vi "rszvl_core_global.vi"() -> ()   [LabVIEW 2014] (continued)
"*WAI"=FALSE}, "Check Status Callback"=""}, {"Level"=2, "Descriptive Name"="Display Window Size", "Class Only"=FALSE, "Data Type"=0, "Access"=2, "Identifier"="RSZVL_ATTR_DISP_WINDOW_SIZE", "Range Table"="rszvl_rngDISPSizeWindow", "Command"="DISP:SIZE", "Read Callback"="", "Write Callback"="", "Range Callback"="", "Check Callback"="", "Rngtable Callback"="", "Coerce Callback"="", "User Callback"="", "Supported Models"="", "Instrument Options"="", "Repeated Capabilities"="", "Restricted Repeated Capabilities"="", "Help"="This attribute switches the measurement window for channel and adjacent-channel power measurements to full screen or half screen.\n\nAvailable Repeated Capabilities:\nNone\n\nRemote-control command(s):\nDISPlay[:WINDow<1|2>]:SIZE LARGe | SMALl", "Flags"={"OPC Wait"=FALSE, "Dont check status"=FALSE, "*WAI"=FALSE}, "Check Status Callback"=""}, {"Level"=2, "Descriptive Name"="Display Color Preset", "Class Only"=FALSE, "Data Type"=4, "Access"=1, "Identifier"="RSZVL_ATTR_DISP_COL_PRESET", "Range Table"="", "Command"="DISP:CMAP:DEF{Default}", "Read Callback"="", "Write Callback"="", "Range Callback"="", "Check Callback"="", "Rngtable Callback"="", "Coerce Callback"="", "User Callback"="", "Supported Models"="", "Instrument Options"="", "Repeated Capabilities"="", "Restricted Repeated Capabilities"="", "Help"="This attribute resets the screen colors of all display items to their default settings. Two default settings DEFault1 and DEFault2 are available. The numeric suffix of CMAP is irrelevant.\n\nAvailable Repeated Capabilities:\nDefault: DEF1,DEF2,DEF3\r\n\nRemote-control command(s):\nDISPlay:CMAP<1 to 27>:DEFault<1|2|3>", "Flags"={"OPC Wait"=FALSE, "Dont check status"=FALSE, "*WAI"=FALSE}, "Check Status Callback"=""}, {"Level"=2, "Descriptive Name"="Display Color Predefined", "Class Only"=FALSE, "Data Type"=0, "Access"=1, "Identifier"="RSZVL_ATTR_DISP_COL_PREDEFINED", "Range Table"="rszvl_rngDISPConfPreDefColour", "Command"="DISP:CMAP{CMAP}:PDEF", "Read Callback"="", "Write Callback"="", "Range Callback"="", "Check Callback"="", "Rngtable Callback"="", "Coerce Callback"="", "User Callback"="", "Supported Models"="", "Instrument Options"="", "Repeated Capabilities"="", "Restricted Repeated Capabilities"="", "Help"="This attribute defines the color table of the instrument using predefined color values. Each numeric suffix of CMAP is assigned one or several graphical elements which can be modified by varying the corresponding color setting.\nThe same assignment as for DISPlay:CMAP<1 to 26>:HSL applies.\n\nAvailable Repeated Capabilities:\nCMAP: CM1,CM2,CM3,CM4,CM5,CM6,CM7,CM8,CM9,CM10,CM11,CM12,CM13,CM14,CM15,CM16,CM17,CM18,CM19,CM20,CM21,CM22,CM23,CM24,CM25,CM26,CM27\r\n\nRemote-control command(s):\nDISPlay:CMAP<1 to 27>:PDEFined BLACk| BLUE| BROWn| GREen|MAGenta| YELLow| WHITe| DGRAy| LGRAy|LBLUe| LGREen| LCYan| LRED| MAGenta", "Flags"={"OPC Wait"=FALSE, "Dont check status"=FALSE, "*WAI"=FALSE}, "Check Status Callback"=""}, {"Level"=2, "Descriptive Name"="Display Log Range", "Class Only"=FALSE, "Data Type"=1, "Access"=2, "Identifier"="RSZVL_ATTR_DISP_LOG_RANGE", "Range Table"="rszvl_rngDISPAmplitudeRang", "Command"="DISP:WIND:TRAC:Y", "Read Callback"="", "Write Callback"="", "Range Callback"="", "Check Callback"="", "Rngtable Callback"="", "Coerce Callback"="", "User Callback"="", "Supported Models"="", "Instrument Options"="", "Repeated Capabilities"="", "Restricted Repeated Capabilities"="", "Help"="This attribute defines the display range of the Y axis (level axis) with logarithmic scaling (DISP:TRAC:Y:SPAC LOG).\nFor linear scaling, (DISP:TRAC:Y:SPAC LIN | PERC) the display range is fixed and cannot be modified.\n\nAvailable Repeated Capabilities:\nNone\n\nRemote-control command(s):\nDISPlay[:WINDow<1|2>]:TRACe<1 to 6>:Y[:SCALe]", "Flags"={"OPC Wait"=FALSE, "Dont check status"=FALSE, "*WAI"=FALSE}, "Check Status Callback"=""}, {"Level"=2, "Descriptive Name"="Display Amplitude Grid Mode", "Class Only"=FALSE, "Data Type"=0, "Access"=2, "Identifier"="RSZVL_ATTR_DISP_AMPLITUDE_GRID_MODE", "Range Table"="rszvl_rngAbsRel", "Command"="DISP:WIND:TRAC:Y:MODE", "Read Callback"="", "Write Callback"="", "Range Callback"="", "Check Callback"="", "Rngtable Callback"="", "Coerce Callback"="", "User Callback"="", "Supported Models"="", "Instrument Options"="", "Repeated Capabilities"="", "Restricted Repeated Capabilities"="", "Help"="This attribute defines the scale type of the Y axis (absolute or relative).\nWhen SYSTem:DISPlay is set to OFF, this command has no immediate effect on the screen. The numeric suffix is irrelevant.\n\nAvailable Repeated Capabilities:\nNone\n\nRemote-control command(s):\nDISPlay[:WINDow<1|2>]:TRACe<1 to 6>:Y[:SCALe]:MODE ABSolute | RELative", "Flags"={"OPC Wait"=FALSE, "Dont check status"=FALSE, "*WAI"=FALSE}, "Check Status Callback"=""}, {"Level"=2, "Descriptive Name"="Display During Single Sweep", "Class Only"=FALSE, "Data Type"=3, "Access"=2, "Identifier"="RSZVL_ATTR_DISP_SINGLE_SWEEP", "Range Table"="", "Command"="INIT:DISP", "Read Callback"="", "Write Callback"="", "Range Callback"="", "Check Callback"="", "Rngtable Callback"="", "Coerce Callback"="", "User Callback"="", "Supported Models"="", "Instrument Options"="", "Repeated Capabilities"="", "Restricted Repeated Capabilities"="", "Help"="This attribute configures the behaviour of the display during a single sweep.\nINITiate:DISPlay OFF means that the display is switched off during the measurement, INITiate:DISPlay ON means that the display is switched on during the measurement.\n\nAvailable Repeated Capabilities:\nNone\n\nRemote-control command(s):\nINITiate:DISPlay ON | OFF", "Flags"={"OPC Wait"=FALSE, "Dont check status"=FALSE, "*WAI"=FALSE}, "Check Status Callback"=""}, {"Level"=2, "Descriptive Name"="Display Update", "Class Only"=FALSE, "Data Type"=3, "Access"=2, "Identifier"="RSZVL_ATTR_DISP_UPDATE", "Range Table"="", "Command"="SYST:DISP:UPD", "Read Callback"="", "Write Callback"="", "Range Callback"="", "Check Callback"="", "Rngtable Callback"="", "Coerce Callback"="", "User Callback"="", "Supported Models"="", "Instrument Options"="", "Repeated Capabilities"="", "Restricted Repeated Capabilities"="", "Help"="This attribute switches on or off the update of all display elements during remote control.\n\nNote: \n(1) The best performance is obtained when the display output is switched off during remote control.\n\nAvailable Repeated Capabilities:\nNone\n\nRemote-control command(s):\nSYSTem:DISPlay:UPDate ON | OFF", "Flags"={"OPC Wait"=FALSE, "Dont check status"=FALSE, "*WAI"=FALSE}, "Check Status Callback"=""}, {"Level"=2, "Descriptive Name"="Configure Display Unit Power", "Class Only"=FALSE, "Data Type"=0, "Access"=2, "Identifier"="RSZVL_ATTR_UNIT_POWER", "Range Table"="rszvl_rngAmplitudeUnitsRangeTable", "Command"="CALC:UNIT:POW", "Read Callback"="", "Write Callback"="", "Range Callback"="", "Check Callback"="", "Rngtable Callback"="", "Coerce Callback"="", "User Callback"="", "Supported Models"="", "Instrument Options"="", "Repeated Capabilities"="", "Restricted Repeated Capabilities"="", "Help"="This attribute selects the unit for power.\n\nAvailable Repeated Capabilities:\nNone\n\nRemote-control command(s):\nCALCulate<1|2>:UNIT:POWer DBM | V | A | W | DBPW | WATT | DBUV | DBMV | VOLT | DBUA | AMPere |DBUV_M | DBUA_M", "Flags"={"OPC Wait"=FALSE, "Dont check status"=FALSE, "*WAI"=FALSE}, "Check Status Callback"=""}, {"Level"=1, "Descriptive Name"="Markers", "Class Only"=TRUE, "Data Type"=0, "Access"=0, "Identifier"="", "Range Table"="", "Command"="", "Read Callback"="", "Write Callback"="", "Range Callback"="", "Check Callback"="", "Rngtable Callback"="", "Coerce Callback"="", "User Callback"="", "Supported Models"="", "Instrument Options"="", "Repeated Capabilities"="", "Restricted Repeated Capabilities"="", "Help"="(1) Marker Amplitude:\nThis attribute queries the measured value of the selected marker. The corresponding marker is activated before or switched to marker mode, if necessary.\nTo obtain a valid query result, a complete sweep with synchronization to the sweep end must be performed between the activation of the marker and the query of the y value. This is only possible in single sweep mode.\nThe query result is output in the unit determined with CALCulate:UNIT.\n\n(2) Marker State:\nThis attribute switches on or off the currently selected marker. If no indication is made, marker 1 is selected automatically. If marker 2, 3 or 4 is selected and used as a delta marker, it is switched to marker mode.\n\n(3) Marker Position:\nThis attribute positions the selected marker to the indicated frequency (span > 0), time (span = 0) or level (APD measurement or CCDF measurement ON). If marker 2, 3 or 4 is selected and used as delta marker, it is switched to marker mode.\n\n(4) Assign Marker to Trace:\nThis attribute assigns the selected marker to the indicated measurement curve. The corresponding trace must be active, i.e. its status must be different from BLANK.\n\n(5) All Markers Off:\nThis attribute switches off all active markers.\n\n(6) Marker Local Oscillator Suppression:\nThis attribute switches the local oscillator suppression for peak search on or off. This setting is valid for all markers and delta markers.\n\n(7) Signal Track State:\nThis attribute switches the signal-track function on or off. The function is independent of the selected marker.\nWith signal track activated, the maximum signal is determined after each frequency sweep and the center frequency is set to the frequency of this signal. Thus with drifting signals the center frequency follows the signal.\n\n(8) Signal Track Bandwidth:\nThis attribute defines the bandwidth around the center frequency within which the largest signal is searched. It is only available in the frequency domain (span > 0).\n\nNote(s):\n(1) The entry of the search bandwidth is only possible if the Signal Track function is switched on (RSZVL_ATTR_SIGNAL_TRACK_STATE).\n\n(9) Signal Track Threshold:\nThis attribute defines the threshold above which the largest signal is searched for. The function is independent of the selected marker. It is only available in the frequency domain (span > 0).\nThe response unit depends on the settings defined with CALC:UNIT.\n\nNote(s):\n(1) The entry of the search threshold is only possible if the Signal Track function is switched on (RSZVL_ATTR_SIGNAL_TRACK_STATE).\n\n(10) Signal Track Trace:\nThis attribute defines the trace on which the largest signal is searched for. The function is independent of the selected marker. It is only available in the frequency domain (span > 0).\n\n(11) Marker Step Size:\nThis command defines the step size of the rotary knob for marker or delta marker value changes. It takes only effect in manual operation. It is available for all base unit measurements with the exception of statistics.\n\n(12) Marker Probability:\nThis command positions the selected marker to the given probability.\n\nNote(s): \n(1) The command is only available with the CCDF measurement switched on. The associated level value can be determined with the CALCulate<1|2>:MARKer<1...4>:X command.\n\n\n(13) Marker Search (Class):\nMarker Search.\n\n(1) Marker Search Right Minimum:\nThis attribute positions the marker to the next higher minimum value to the right of the current value (i.e. in ascending X direction) on the corresponding trace.\n\n(2) Marker Search Left Minimum:\nThis attribute positions the marker to the next higher minimum value to the left of the current value (i.e. in descending X direction) on the corresponding trace.\n\n(3) Marker Search Peak Maximum:\nThis attribute positions the marker to the current maximum value of the corresponding trace. The corresponding marker is activated first or switched to the marker mode.\nNote: If no maximum value is found on the trace (level spacing to adjacent values < peak excursion), an execution error (error eode: -200) is produced.\n\n(4) Marker Search Peak Next Maximum:\nThis attribute positions the marker to the next smaller maximum value of the corresponding trace.\n\n(5) Marker Search Peak Right Maximum:\nThis attribute positions the marker to the next smaller maximum value to the right of the current value (i.e. in ascending X values) on the corresponding trace.\n\n(6) Marker Search Peak Left Maximum:\nThis attribute positions the marker to the next smaller maximum value to the left of the current value (i.e. in descending X values) on the trace.\n\n(7) Marker Search Peak Minimum:\nThis attribute positions the marker to the current minimum value of the corresponding trace. The corresponding marker is activated first or switched to marker mode, if necessary.\n\n(8) Marker Search Next Minimum:\nThis attribute positions the marker to the next higher minimum value of the corresponding trace.\n\n(9) Marker Search Peak Maximum Auto:\nThis attribute switches an automatic maximum peak search for marker 1 at the end of each particular sweep on and off. The actual marker search limit settings (LEFT LIMIT, RIGHT LIMIT, THRESHOLD, EXCLUDE LO) are taken into account.\n\n(10) Marker Search Minimum Auto:\nThis attribute switches an automatic minimum peak search for marker 1 at the end of each particular sweep on and off. The actual marker search limit settings (LEFT LIMIT, RIGHT LIMIT, THRESHOLD, EXCLUDE LO) are taken into account.\n\n(14) Marker Search Configuration (Class):\nConfigures marker search parameters.\n\n(1) Marker Threshold State:\nThis attribute switches on or off the threshold line. The unit depends on the setting performed with CALC:UNIT.\n\n(2) Marker Threshold:\nThis attribute defines the threshold value for the maximum/minimum search of markers with marker search functions MAX PEAK, NEXT PEAK, etc. The associated display line is automatically switched on.\n\n(3) Marker Peak Excursion:\nThis attribute defines the peak excursion., i.e. the spacing below a trace maximum which must be attained before a new maximum is recognized, or the spacing above a trace minimum which must be attained before a new minimum is recognized. The set value is valid for all markers and delta markers. The unit depends on the selected operating mode.\n\n(4) Marker Search Limits State:\nThis attribute switches between a limited (ON) and unlimited (OFF) search range. The function is independent of the selection of a marker.\n\n(5) Marker Search Limits Left:\nThis attribute sets the left limit of the search range for markers and delta markers. Depending on the x axis domain the indicated value defines a frequency (span > 0) or time (span = 0). The function is independent of the selection of a marker.\n\n(6) Marker Search Limits Right:\nThis attribute sets the right limit of the search range for markers and delta markers. Depending on the x axis domain the indicated value defines a frequency (span > 0) or time (span = 0). The function is independent of the selection of a marker.\n\n\n\n(15) Marker Functions (Class):\nMarker Functions.\n\n(1) Marker Peak List Count:\nThis attribute searches the selected trace for the indicated number of maxima. The number of maxima found depends on the waveform and value set for the Peak Excursion parameter, however, a maximum number of 50 maxima are determined. Only the signals which exceed their surrounding values at least by the value indicated by the peak excursion parameter will be recognized as maxima. Therefore, the number of maxima found is not automatically the same as the number of maxima desired.\n\n(2) Marker Peak List Found:\nThis attribute reads out the number of maxima found during the search. If no search for maxima has been performed, 0 is returned.\n\n(3) Marker Peak List Sort:\nThis attribute sets the sort mode for the search for maxima.\n\n(4) Marker Zoom:\nThis attribute defines the range to be zoomed around marker 1. Marker 1 is activated first, if necessary.\nThe subsequent frequency sweep is stopped at the marker position and the frequency of the signal is counted. This frequency becomes the new center frequency, and the zoomed span is set. In order to recognize the end of the operation the synchronization to the sweep end should be activated. This is only possible in single sweep mode.\n\n(5) Marker Demodulation State:\nThis attribute switches on or off the audio demodulator when the indicated marker is reached. In the frequency domain (span > 0) the hold time can be defined at the corresponding marker position with RSZVL_ATTR_MARKER_DEMOD_HOLDOFF.\nIn the time domain (span = 0) the demodulation is permanently active.\n\n(6) Marker Demodulation Type:\nThis attribute selects the demodulation type for the audio demodulator.\n\n(7) Marker Demodulation Holdoff:\nThis attribute defines the hold time at the marker position for the demodulation in the frequency domain (span > 0).\n\n(8) Marker Demodulation Continuous:\nThis attribute switches on or off the continuous demodulation in the frequency domain (span >0). Thus acoustic monitoring of the signals can be performed in the frequency domain. The function does not depend on the selected marker.\n\n(9) Marker To Center:\nThis attribute sets the center frequency equal to the frequency of the indicated marker.\nIf marker 2, 3 or 4 is selected and used as delta marker, it is switched to the marker mode.\n\n(10) Marker To Step Width:\nThis attribute sets the step width of the center frequency to the X value of the current marker. If marker 2, 3 or 4 is selected and used as delta marker, it is switched to the marker mode.\n\n(11) Marker To Reference:\nThis attribute sets the reference level to the power measured by the indicated marker. If marker 2, 3 or 4 is selected and used as delta marker, it is switched to marker mode.\n\n(12) Marker Fixed Reference State:\nThis attribute switches the relative measurement to a fixed reference value on or off. Marker 1 will be activated previously and a peak search will be performed, if necessary. If marker 1 is activated, its position becomes the reference point for the measurement. The reference point can then be modified with commands CALCulate:DELTamarker:FUNCtion:FIXed:RPOint:X and to :RPOint:Y independently of the position of marker 1 and of a trace. It is valid for all delta markers as long as the function is active.\n\n(13) Marker Fixed Ref Point Level:\nThis attribute defines a new reference point level for all delta markers for a measurement with fixed reference point.\n(CALCulate:DELTamarker:FUNCtion:FIXed:STATe ON).\nFor phase-noise measurements (CALCulate:DELTamarker:FUNCtion:PNOise:STATe ON), the command defines a new reference point level for delta marker 2.\n\n(14) Marker Fixed Ref Point Level Offset:\nThis attribute defines an additional level offset for the measurement with fixed reference value (CALCulate:DELTamarker:FUNCtion:FIXed:STATe ON). For this measurement, the offset is included in the display of all delta markers.\nFor phase-noise measurements (CALCulate:DELTamarker:FUNCtion:PNOise:STATe ON), the command defines an additional level offset which is included in the display of delta marker 2.\n\n(15) Marker Fixed Ref Point Frequency:\nThis attribute defines a new reference frequency (span > 0) or time (span = 0) for all delta markers for a measurement with fixed reference value (CALCulate:DELTamarker:FUNCtion:FIXed:STATe ON).\nFor phase-noise measurements (CALCulate:DELTamarker:FUNCtion:PNOise:STATe ON), the command defines a new reference frequency or time for delta marker 2.\n\n(16) Marker Fixed Ref Point Peak Search:\nThis attribute sets the reference point level for all delta markers for a measurement with fixed reference point (CALC:DELT:FUNC:FIX:STAT ON) to the peak of the selected trace.\n\n\n\n(16) Delta Marker (Class):\nDelta Marker attributes configuration.\n\n(1) Delta Marker State:\nThis attribute switches on and off the delta marker when delta marker 1 is selected. The corresponding marker becomes the delta marker when delta marker 2 to 4 is selected. If the corresponding marker is not activated, it will be activated and positioned on  the maximum of the measurement curve.\n\n(2) Delta Marker Mode:\nThis attribute switches between relative and absolute frequency input of the delta marker (or time with span = 0). It affects all delta markers.\nRepeated capabilitiy Delta Marker are used to prevent switching On Delta Marker 1, if the user uses Delta Marker 2.\n\n(3) Delta Marker Position:\nThis attribute positions the selected delta marker to the indicated frequency (span > 0), time (span = 0) or level (APD measurement = ON or CCDFmeasurement = ON). The input is in absolute values or relative to marker 1 depending on the attribute RSZVL_ATTR_REFERENCE_MARKER_MODE. If Reference Fixed measurement (CALCulate:DELTamarker:FUNCtion:FIXed:STATe ON) is active, relative values refer to the reference position are entered. The query always returns absolute values.\n\n(4) Delta Marker Relative Position:\nThis attribute queries the frequency (span > 0) or time (span = 0) of the selected delta marker relative to marker 1 or to the reference position ( for CALCulate:DELTamarker:FUNCtion:FIXed:STATe ON). The attribute activates the corresponding delta marker, if necessary.\n\n(5) Delta Marker Amplitude:\nThis attribute queries the measured value of the selected delta marker. The corresponding delta marker will be activated, if necessary. The output is always a relative value referred to marker 1 or to the reference position (reference fixed active).\n\n(6) Delta Marker Assign Trace:\nThis attribute assigns the selected delta marker to the indicated measurement curve. The selected measurement curve must be active, i.e. its state must be different from BLANK.\n\n(7) Delta Marker All Off:\nThis attribute switches off all active delta markers (screen A or screen B).\n\n(17) Delta Marker Search (Class):\nDelta marker search.\n\n(1) Delta Marker Peak:\nThis attribute positions the delta marker to the current maximum value on the measured curve. If necessary, the corresponding delta marker will be activated first.\n\n(2) Delta Marker Peak Next:\nThis attribute positions the delta marker to the next smaller maximum value on the measured curve. The corresponding delta marker will be activated first, if necessary.\n\n(3) Delta Marker Peak Next Right:\nThis attribute positions the delta marker to the next smaller maximum value to the right of the current value (i.e. ascending X values). The corresponding delta marker is activated first, if necessary.\n\n(4) Delta Marker Peak Next Left:\nThis attribute positions the delta marker to the next smaller maximum value to the left of the current value (i.e. descending X values). The corresponding delta marker will be activated first, if necessary.\n\n(5) Delta Marker Minimum:\nThis attribute positions the delta marker to the current minimum value on the measured crve. The corresponding delta marker will be activated first, if necessary.\n\n(6) Delta Marker Minimum Next:\nThis attribute positions the delta marker to the next higher minimum value of the measured curve. The corresponding delta marker will be activated first, if necessary.\n\n(7) Delta Marker Minimum Next Right:\nThis attribute positions the delta marker to the next higher minimum value to the right of the current value (i.e. ascending X values). The corresponding delta marker will be activated first, if necessary.\n\n(8) Delta Marker Minimum Next Left:\nThis attribute positions the delta marker to the next higher minimum value to the left of the current value (i.e. descending X values). The corresponding delta marker will be activated first, if necessary.", "Flags"={"OPC Wait"=FALSE, "Dont check status"=FALSE, "*WAI"=FALSE}, "Check Status Callback"=""}, {"Level"=2, "Descriptive Name"="Marker Amplitude", "Class Only"=FALSE, "Data Type"=1, "Access"=0, "Identifier"="RSZVL_ATTR_MARKER_AMPLITUDE", "Range Table"="", "Command"="CALC:MARK{Marker}:Y?", "Read Callback"="", "Write Callback"="", "Range Callback"="", "Check Callback"="", "Rngtable Callback"="", "Coerce Callback"="", "User Callback"="", "Supported Models"="", "Instrument Options"="", "Repeated Capabilities"="", "Restricted Repeated Capabilities"="", "Help"="This attribute queries the measured value of the selected marker. The corresponding marker is activated before or switched to marker mode, if necessary.\nTo obtain a valid query result, a complete sweep with synchronization to the sweep end must be performed between the activation of the marker and the query of the y value. This is only possible in single sweep mode.\nThe query result is output in the unit determined with CALCulate:UNIT.\n\nAvailable Repeated Capabilities:\nMarker: M1,M2,M3,M4\r\n\nRemote-control command(s):\nCALCulate<1|2>:MARKer<1 to 4>:Y?", "Flags"={"OPC Wait"=FALSE, "Dont check status"=FALSE, "*WAI"=FALSE}, "Check Status Callback"=""}, {"Level"=2, "Descriptive Name"="Marker State", "Class Only"=FALSE, "Data Type"=3, "Access"=2, "Identifier"="RSZVL_ATTR_MARKER_ENABLED", "Range Table"="", "Command"="CALC:MARK{Marker}", "Read Callback"="", "Write Callback"="", "Range Callback"="", "Check Callback"="", "Rngtable Callback"="", "Coerce Callback"="", "User Callback"="", "Supported Models"="", "Instrument Options"="", "Repeated Capabilities"="", "Restricted Repeated Capabilities"="", "Help"="This attribute switches on or off the currently selected marker. If no indication is made, marker 1 is selected automatically. If marker 2, 3 or 4 is selected and used as a delta marker, it is switched to marker mode.\n\nAvailable Repeated Capabilities:\nMarker: M1,M2,M3,M4\r\n\nRemote-control command(s):\nCALCulate<1|2>:MARKer<1 to 4>[:STATe]", "Flags"={"OPC Wait"=FALSE, "Dont check status"=FALSE, "*WAI"=FALSE}, "Check Status Callback"=""}, {"Level"=2, "Descriptive Name"="Marker Position", "Class Only"=FALSE, "Data Type"=1, "Access"=2, "Identifier"="RSZVL_ATTR_MARKER_POSITION", "Range Table"="", "Command"="CALC:MARK{Marker}:X", "Read Callback"="", "Write Callback"="", "Range Callback"="", "Check Callback"="", "Rngtable Callback"="", "Coerce Callback"="", "User Callback"="", "Supported Models"="", "Instrument Options"="", "Repeated Capabilities"="", "Restricted Repeated Capabilities"="", "Help"="This attribute positions the selected marker to the indicated frequency (span > 0), time (span = 0) or level (APD measurement or CCDF measurement ON). If marker 2, 3 or 4 is selected and used as delta marker, it is switched to marker mode.\n\nAvailable Repeated Capabilities:\nMarker: M1,M2,M3,M4\r\n\nRemote-control command(s):\nCALCulate<1|2>:MARKer<1 to 4>:X", "Flags"={"OPC Wait"=FALSE, "Dont check status"=FALSE, "*WAI"=FALSE}, "Check Status Callback"=""}, {"Level"=2, "Descriptive Name"="Assign Marker to Trace", "Class Only"=FALSE, "Data Type"=0, "Access"=2, "Identifier"="RSZVL_ATTR_MARKER_TRACE", "Range Table"="rszvl_rngTrace", "Command"="CALC:MARK{Marker}:TRAC", "Read Callback"="", "Write Callback"="", "Range Callback"="", "Check Callback"="", "Rngtable Callback"="", "Coerce Callback"="", "User Callback"="", "Supported Models"="", "Instrument Options"="", "Repeated Capabilities"="", "Restricted Repeated Capabilities"="", "Help"="This attribute assigns the selected marker to the indicated measurement curve. The corresponding trace must be active, i.e. its status must be different from BLANK.\n\nAvailable Repeated Capabilities:\nMarker: M1,M2,M3,M4\r\n\nRemote-control command(s):\nCALCulate<1|2>:MARKer<1 to 4>:TRACe", "Flags"={"OPC Wait"=FALSE, "Dont check status"=FALSE, "*WAI"=FALSE}, "Check Status Callback"=""}, {"Level"=2, "Descriptive Name"="All Markers Off", "Class Only"=FALSE, "Data Type"=4, "Access"=1, "Identifier"="RSZVL_ATTR_MARKER_AOFF", "Range Table"="", "Command"="CALC:MARK:AOFF", "Read Callback"="", "Write Callback"="", "Range Callback"="", "Check Callback"="", "Rngtable Callback"="", "Coerce Callback"="", "User Callback"="", "Supported Models"="", "Instrument Options"="", "Repeated Capabilities"="", "Restricted Repeated Capabilities"="", "Help"="This attribute switches off all active markers.\n\nAvailable Repeated Capabilities:\nNone\n\nRemote-control command(s):\nCALCulate<1|2>:MARKer<1 to 4>:AOFF", "Flags"={"OPC Wait"=FALSE, "Dont check status"=FALSE, "*WAI"=FALSE}, "Check Status Callback"=""}, {"Level"=2, "Descriptive Name"="Marker Local Oscillator Suppression", "Class Only"=FALSE, "Data Type"=3, "Access"=2, "Identifier"="RSZVL_ATTR_MARKER_LOEX", "Range Table"="", "Command"="CALC:MARK:LOEX", "Read Callback"="", "Write Callback"="", "Range Callback"="", "Check Callback"="", "Rngtable Callback"="", "Coerce Callback"="", "User Callback"="", "Supported Models"="", "Instrument Options"="", "Repeated Capabilities"="", "Restricted Repeated Capabilities"="", "Help"="This attribute switches the local oscillator suppression for peak search on or off. This setting is valid for all markers and delta markers.\n\nAvailable Repeated Capabilities:\nNone\n\nRemote-control command(s):\nCALCulate<1|2>:MARKer<1 to 4>:LOEXclude ON | OFF", "Flags"={"OPC Wait"=FALSE, "Dont check status"=FALSE, "*WAI"=FALSE}, "Check Status Callback"=""}, {"Level"=2, "Descriptive Name"="Signal Track State", "Class Only"=FALSE, "Data Type"=3, "Access"=2, "Identifier"="RSZVL_ATTR_SIGNAL_TRACK_ENABLED", "Range Table"="", "Command"="CALC:MARK:FUNC:STR", "Read Callback"="", "Write Callback"="", "Range Callback"="", "Check Callback"="", "Rngtable Callback"="", "Coerce Callback"="", "User Callback"="", "Supported Models"="", "Instrument Options"="", "Repeated Capabilities"="", "Restricted Repeated Capabilities"="", "Help"="This attribute switches the signal-track function on or off. The function is independent of the selected marker.\nWith signal track activated, the maximum signal is determined after each frequency sweep and the center frequency is set to the frequency of this signal. Thus with drifting signals the center frequency follows the signal.\n\nAvailable Repeated Capabilities:\nNone\n\nRemote-control command(s):\nCALCulate<1|2>:MARKer<1 to 4>:FUNCtion:STRack[:STATe] ON | OFF", "Flags"={"OPC Wait"=FALSE, "Dont check status"=FALSE, "*WAI"=FALSE}, "Check Status Callback"=""}, {"Level"=2, "Descriptive Name"="Signal Track Bandwidth", "Class Only"=FALSE, "Data Type"=1, "Access"=2, "Identifier"="RSZVL_ATTR_SIGNAL_TRACK_BWID", "Range Table"="", "Command"="CALC:MARK:FUNC:STR:BWID", "Read Callback"="", "Write Callback"="", "Range Callback"="", "Check Callback"="", "Rngtable Callback"="", "Coerce Callback"="", "User Callback"="", "Supported Models"="", "Instrument Options"="", "Repeated Capabilities"="", "Restricted Repeated Capabilities"="", "Help"="This attribute defines the bandwidth around the center frequency within which the largest signal is searched. It is only available in the frequency domain (span > 0).\n\nNote(s):\n(1) The entry of the search bandwidth is only possible if the Signal Track function is switched on (RSZVL_ATTR_SIGNAL_TRACK_STATE).\n\nAvailable Repeated Capabilities:\nNone\n\nRemote-control command(s):\nCALCulate<1|2>:MARKer<1 to 4>:FUNCtion:STRack:BWIDth", "Flags"={"OPC Wait"=FALSE, "Dont check status"=FALSE, "*WAI"=FALSE}, "Check Status Callback"=""}, {"Level"=2, "Descriptive Name"="Signal Track Threshold", "Class Only"=FALSE, "Data Type"=1, "Access"=2, "Identifier"="RSZVL_ATTR_SIGNAL_TRACK_THRESHOLD", "Range Table"="rszvl_rngSignalTrackThreshold", "Command"="CALC:MARK:FUNC:STR:THR", "Read Callback"="", "Write Callback"="", "Range Callback"="", "Check Callback"="", "Rngtable Callback"="", "Coerce Callback"="", "User Callback"="", "Supported Models"="", "Instrument Options"="", "Repeated Capabilities"="", "Restricted Repeated Capabilities"="", "Help"="This attribute defines the threshold above which the largest signal is searched for. The function is independent of the selected marker. It is only available in the frequency domain (span > 0).\nThe response unit depends on the settings defined with CALC:UNIT.\n\nNote(s):\n(1) The entry of the search threshold is only possible if the Signal Track function is switched on (RSZVL_ATTR_SIGNAL_TRACK_STATE).\n\nAvailable Repeated Capabilities:\nNone\n\nRemote-control command(s):\nCALCulate<1|2>:MARKer<1 to 4>:FUNCtion:STRack:THReshold", "Flags"={"OPC Wait"=FALSE, "Dont check status"=FALSE, "*WAI"=FALSE}, "Check Status Callback"=""}, {"Level"=2, "Descriptive Name"="Signal Track Trace", "Class Only"=FALSE, "Data Type"=0, "Access"=2, "Identifier"="RSZVL_ATTR_SIGNAL_TRACK_TRACE", "Range Table"="rszvl_rngTrace", "Command"="CALC:MARK:FUNC:STR:TRAC", "Read Callback"="", "Write Callback"="", "Range Callback"="", "Check Callback"="", "Rngtable Callback"="", "Coerce Callback"="", "User Callback"="", "Supported Models"="", "Instrument Options"="", "Repeated Capabilities"="", "Restricted Repeated Capabilities"="", "Help"="This attribute defines the trace on which the largest signal is searched for. The function is independent of the selected marker. It is only available in the frequency domain (span > 0).\n\nAvailable Repeated Capabilities:\nNone\n\nRemote-control command(s):\nCALCulate<1|2>:MARKer<1 to 4>:FUNCtion:STRack:TRACe", "Flags"={"OPC Wait"=FALSE, "Dont check status"=FALSE, "*WAI"=FALSE}, "Check Status Callback"=""}, {"Level"=2, "Descriptive Name"="Marker Step Size", "Class Only"=FALSE, "Data Type"=0, "Access"=2, "Identifier"="RSZVL_ATTR_MARKER_STEP_SIZE", "Range Table"="rszvl_rngMarkerStepSize", "Command"="CALC:MARK:X:SSIZ", "Read Callback"="", "Write Callback"="", "Range Callback"="", "Check Callback"="", "Rngtable Callback"="", "Coerce Callback"="", "User Callback"="", "Supported Models"="", "Instrument Options"="", "Repeated Capabilities"="", "Restricted Repeated Capabilities"="", "Help"="This command defines the step size of the rotary knob for marker or delta marker value changes. It takes only effect in manual operation. It is available for all base unit measurements with the exception of statistics.\n\nAvailable Repeated Capabilities:\nNone\n\nRemote-control command(s):\nCALCulate<1|2>:MARKer<1...4>:X:SSIZe", "Flags"={"OPC Wait"=FALSE, "Dont check status"=FALSE, "*WAI"=FALSE}, "Check Status Callback"=""}, {"Level"=2, "Descriptive Name"="Marker Probability", "Class Only"=FALSE, "Data Type"=1, "Access"=2, "Identifier"="RSZVL_ATTR_MARKER_PROBABILITY", "Range Table"="rszvl_rngPct", "Command"="CALC:MARK{Marker}:Y:PERC", "Read Callback"="", "Write Callback"="", "Range Callback"="", "Check Callback"="", "Rngtable Callback"="", "Coerce Callback"="", "User Callback"="", "Supported Models"="", "Instrument Options"="", "Repeated Capabilities"="", "Restricted Repeated Capabilities"="", "Help"="This command positions the selected marker to the given probability.\n\nNote(s): \n(1) The command is only available with the CCDF measurement switched on. The associated level value can be determined with the CALCulate<1|2>:MARKer<1...4>:X command.\n\nAvailable Repeated Capabilities:\nMarker: M1,M2,M3,M4\r\n\nRemote-control command(s):\nCALCulate<1|2>:MARKer<1...4>:Y:PERCent", "Flags"={"OPC Wait"=FALSE, "Dont check status"=FALSE, "*WAI"=FALSE}, "Check Status Callback"=""}, {"Level"=2, "Descriptive Name"="Marker Search", "Class Only"=TRUE, "Data Type"=0, "Access"=0, "Identifier"="", "Range Table"="", "Command"="", "Read Callback"="", "Write Callback"="", "Range Callback"="", "Check Callback"="", "Rngtable Callback"="", "Coerce Callback"="", "User Callback"="", "Supported Models"="", "Instrument Options"="", "Repeated Capabilities"="", "Restricted Repeated Capabilities"="", "Help"="Marker Search.\n\n(1) Marker Search Right Minimum:\nThis attribute positions the marker to the next higher minimum value to the right of the current value (i.e. in ascending X direction) on the corresponding trace.\n\n(2) Marker Search Left Minimum:\nThis attribute positions the marker to the next higher minimum value to the left of the current value (i.e. in descending X direction) on the corresponding trace.\n\n(3) Marker Search Peak Maximum:\nThis attribute positions the marker to the current maximum value of the corresponding trace. The corresponding marker is activated first or switched to the marker mode.\nNote: If no maximum value is found on the trace (level spacing to adjacent values < peak excursion), an execution error (error eode: -200) is produced.\n\n(4) Marker Search Peak Next Maximum:\nThis attribute positions the marker to the next smaller maximum value of the corresponding trace.\n\n(5) Marker Search Peak Right Maximum:\nThis attribute positions the marker to the next smaller maximum value to the right of the current value (i.e. in ascending X values) on the corresponding trace.\n\n(6) Marker Search Peak Left Maximum:\nThis attribute positions the marker to the next smaller maximum value to the left of the current value (i.e. in descending X values) on the trace.\n\n(7) Marker Search Peak Minimum:\nThis attribute positions the marker to the current minimum value of the corresponding trace. The corresponding marker is activated first or switched to marker mode, if necessary.\n\n(8) Marker Search Next Minimum:\nThis attribute positions the marker to the next higher minimum value of the corresponding trace.\n\n(9) Marker Search Peak Maximum Auto:\nThis attribute switches an automatic maximum peak search for marker 1 at the end of each particular sweep on and off. The actual marker search limit settings (LEFT LIMIT, RIGHT LIMIT, THRESHOLD, EXCLUDE LO) are taken into account.\n\n(10) Marker Search Minimum Auto:\nThis attribute switches an automatic minimum peak search for marker 1 at the end of each particular sweep on and off. The actual marker search limit settings (LEFT LIMIT, RIGHT LIMIT, THRESHOLD, EXCLUDE LO) are taken into account.", "Flags"={"OPC Wait"=FALSE, "Dont check status"=FALSE, "*WAI"=FALSE}, "Check Status Callback"=""}, {"Level"=3, "Descriptive Name"="Marker Search Right Minimum", "Class Only"=FALSE, "Data Type"=4, "Access"=1, "Identifier"="RSZVL_ATTR_MARKER_SEARCH_MIN_RIGHT", "Range Table"="", "Command"="CALC:MARK{Marker}:MIN:RIGH", "Read Callback"="", "Write Callback"="", "Range Callback"="", "Check Callback"="", "Rngtable Callback"="", "Coerce Callback"="", "User Callback"="", "Supported Models"="", "Instrument Options"="", "Repeated Capabilities"="", "Restricted Repeated Capabilities"="", "Help"="This attribute positions the marker to the next higher minimum value to the right of the current value (i.e. in ascending X direction) on the corresponding trace.\n\nNote: If no next higher minimum value is found on the trace (level spacing to adjacent values < peak excursion), an execution error (error code: -200) is produced.\n\nAvailable Repeated Capabilities:\nMarker: M1,M2,M3,M4\r\n\nRemote-control command(s):\nCALCulate<1|2>:MARKer<1 to 4>:MINimum:RIGHt", "Flags"={"OPC Wait"=FALSE, "Dont check status"=FALSE, "*WAI"=FALSE}, "Check Status Callback"=""}, {"Level"=3, "Descriptive Name"="Marker Search Left Minimum", "Class Only"=FALSE, "Data Type"=4, "Access"=1, "Identifier"="RSZVL_ATTR_MARKER_SEARCH_MIN_LEFT", "Range Table"="", "Command"="CALC:MARK{Marker}:MIN:LEFT", "Read Callback"="", "Write Callback"="", "Range Callback"="", "Check Callback"="", "Rngtable Callback"="", "Coerce Callback"="", "User Callback"="", "Supported Models"="", "Instrument Options"="", "Repeated Capabilities"="", "Restricted Repeated Capabilities"="", "Help"="This attribute positions the marker to the next higher minimum value to the left of the current value (i.e. in descending X direction) on the corresponding trace.\n\nNote: If no next higher minimum value is found on the trace (level spacing to adjacent values < peak excursion), an execution error (error code: -200) is produced.\n\nAvailable Repeated Capabilities:\nMarker: M1,M2,M3,M4\r\n\nRemote-control command(s):\nCALCulate<1|2>:MARKer<1 to 4>:MINimum:LEFT", "Flags"={"OPC Wait"=FALSE, "Dont check status"=FALSE, "*WAI"=FALSE}, "Check Status Callback"=""}, {"Level"=3, "Descriptive Name"="Marker Search Peak Maximum", "Class Only"=FALSE, 
